vi "MeasureIVandCap.vi"(0 ".NET Refnum in":refnum<k24>, 1 ".NET Refnum":refnum<k24>, 2 "Junction Name":string, 7 "appended path":path, 9 "Numeric":dbl, 12 "new file path (Not A Path if cancelled)":path, 13 "UiDefinition":T1, 14 "Function":string) -> (15 "error out":errorcluster)   [LabVIEW 2020]
uses:
  D:/LabviewDXFViewer/LabviewDXFViewer/bin/Release/LabviewDXFViewer.exe
  LabviewDXFViewer/bin/Release/LabviewDXFViewer.exe
  UIReferences.ctl
  <vilib>/Utility/file.llb/Write Delimited Spreadsheet (DBL).vi
  <vilib>/Utility/file.llb/Write Delimited Spreadsheet (string).vi
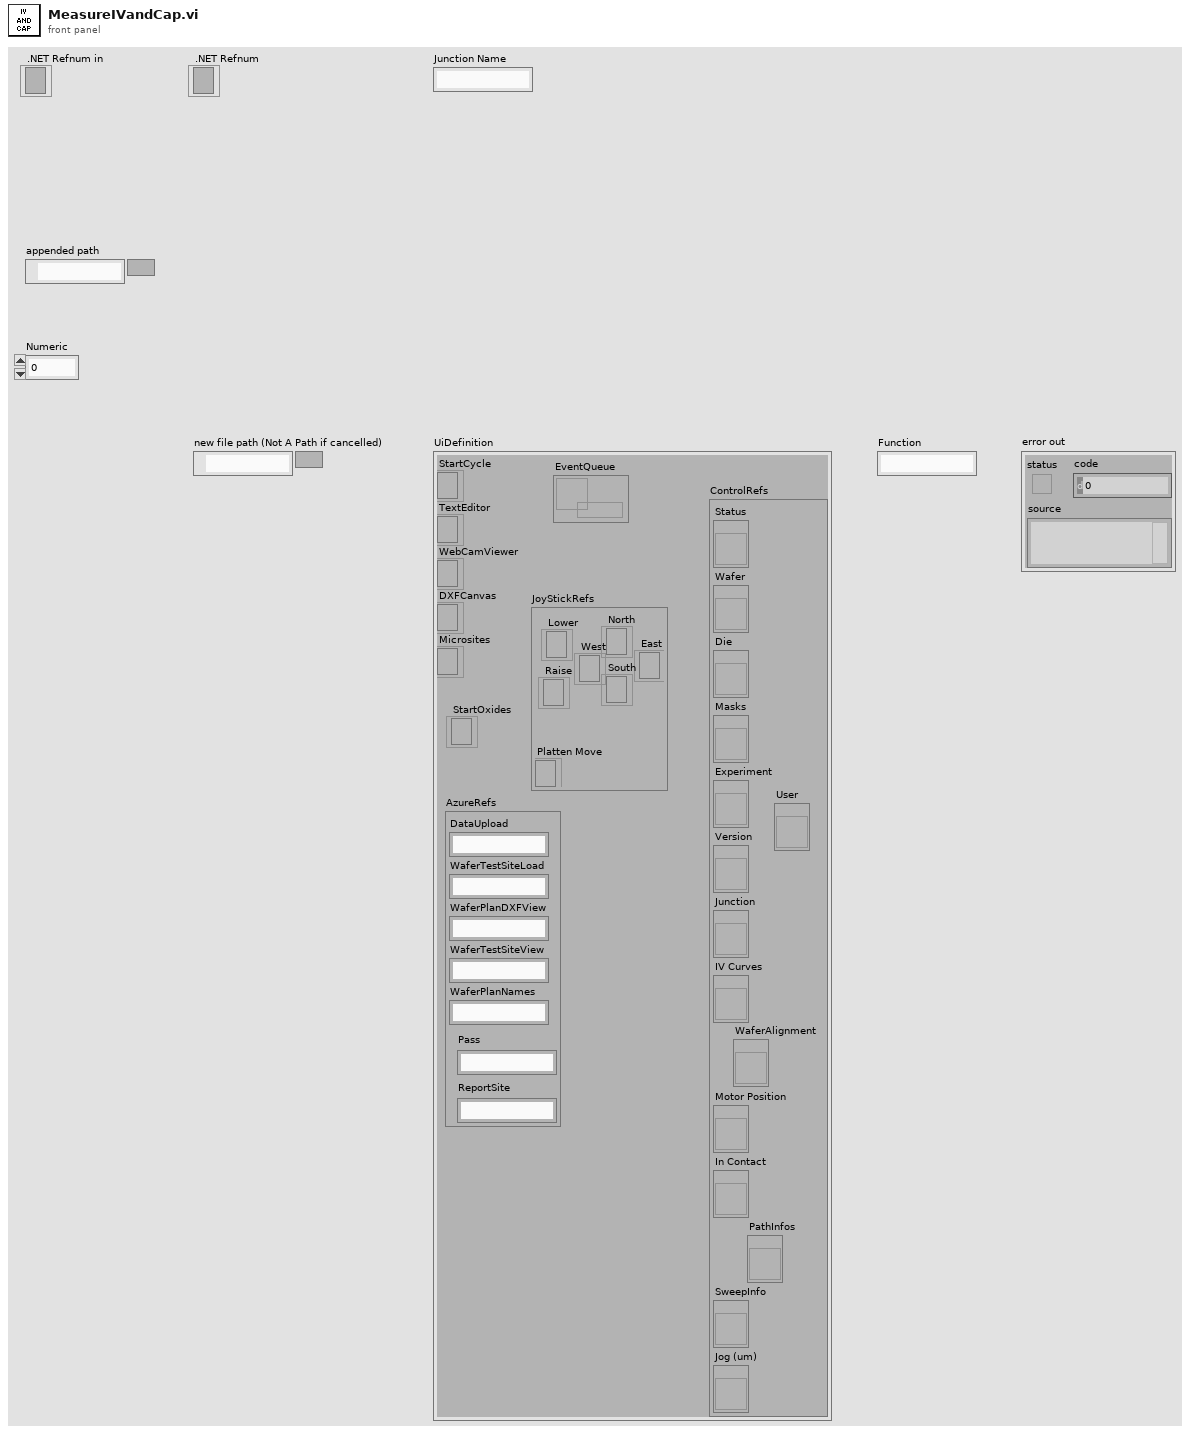
[diagram p1: front panel]
types:
  T1 = typedef "UIReferences.ctl" = cluster{"StartCycle":refnum<k24>, "TextEditor":refnum<k24>, "WebCamViewer":refnum<k24>, "DXFCanvas":refnum<k24>, "Microsites":refnum<k24>, "JoyStickRefs":cluster{"North":refnum<k24>, "Lower":refnum<k24>, "Raise":refnum<k24>, "Platten Move":refnum<k24>, "West":refnum<k24>, "East":refnum<k24>, "South":refnum<k24>}, "AzureRefs":cluster{"DataUpload":string, "WaferTestSiteLoad":string, "WaferPlanDXFView":string, "WaferTestSiteView":string, "WaferPlanNames":string, "Pass":string, "ReportSite":string}, "ControlRefs":cluster{"Status":refnum<vi>, "Wafer":refnum<vi>, "Die":refnum<vi>, "Masks":refnum<vi>, "Experiment":refnum<vi>, "Version":refnum<vi>, "Junction":refnum<vi>, "IV Curves":refnum<vi>, "Motor Position":refnum<vi>, "In Contact":refnum<vi>, "SweepInfo":refnum<vi>, "Jog (um)":refnum<vi>, "PathInfos":refnum<vi>, "User":refnum<vi>, "WaferAlignment":refnum<vi>}, "EventQueue":refnum<queue>, "StartOxides":refnum<k24>}
  T2 = typedef "CapacitanceInfos.ctl" = cluster{"Conductance":dbl, "CapacitanceIV":dbl, "Intercept":dbl, "CapacitanceSW":dbl, "Sum":dbl, "CapacitanceInfos":T3[], "CapacitancePhase":dbl, "dC/dV":dbl, "Function":string}
  T3 = typedef "CapacitanceRecord.ctl" = cluster{"Freq":dbl, "Vpp":dbl, "PhaseS":dbl, "Irms":dbl, "PhaseC":dbl, "Theta":dbl, "VDrive":dbl, "Capacitance":dbl, "Other":dbl}
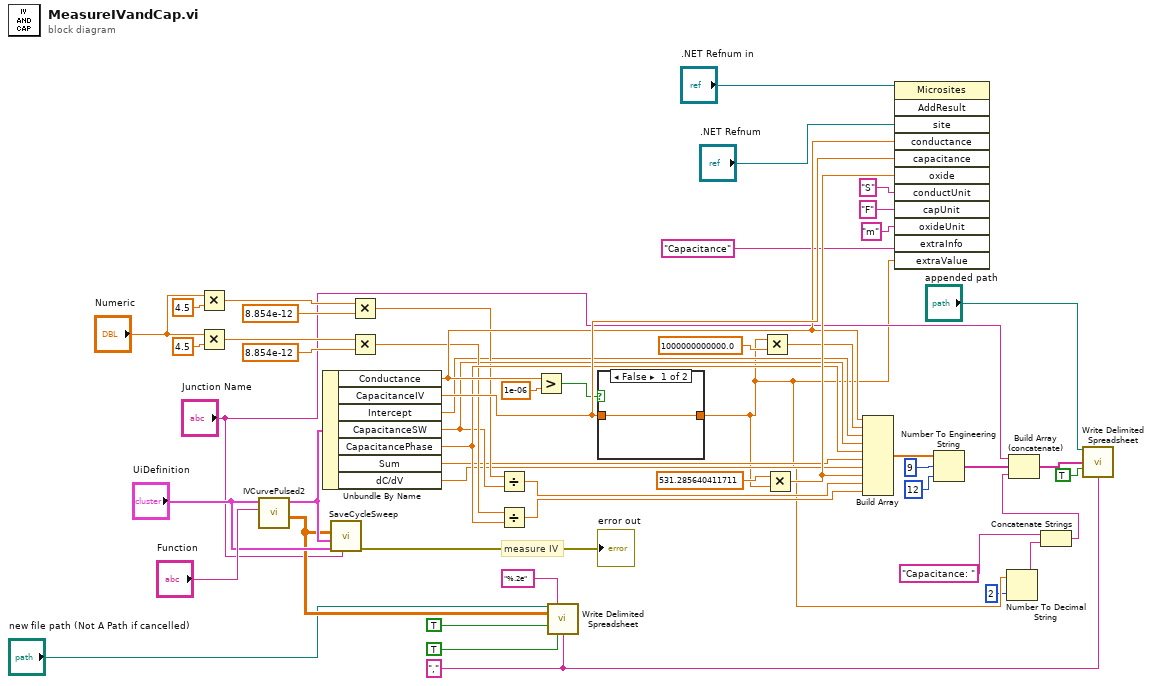
[diagram p0: block diagram]
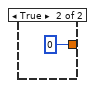
[diagram p2: hidden frame]
diagram:
  w7 = "," ("delimiter (\\t)")
  # "measure IV"
  n1 = Multiply(x="Numeric", y=4.5) -> (x*y=w28:dbl)
  n2 = Multiply(x="Numeric", y=4.5) -> (x*y=w34:dbl)
  n3 = call "IVCurvePulsed2.vi"("Program"="Function", "UiDefinition"="UiDefinition") -> ("appended array"=w18:dbl[][], "InfoCluster"=w48:T2)  [unwired: 8 in]
  n4 = Unbundle By Name(w48) -> ("Conductance"=w50:dbl, "CapacitanceIV"=w51:dbl, "Intercept"=w22:dbl, "CapacitanceSW"=w31:dbl, "CapacitancePhase"=w38:dbl, "Sum"=w23:dbl, "dC/dV"=w24:dbl)
  n5 = call "SaveCycleSweep.vi"("JunctionName"="Junction Name", "UiDefinition 2"="UiDefinition", "InfoCluster"=w48, "appended array"=w18) -> ("error out"=→"error out":errorcluster)  [unwired: 7 in]
  n6 = Multiply(x=w28, y=8.854e-12) -> (x*y=w30:dbl)
  n7 = Multiply(x=w34, y=8.854e-12) -> (x*y=w36:dbl)
  n8 = Divide(x=w30, y=w31) -> (x/y=w32:dbl)
  n9 = Divide(x=w36, y=w38) -> (x/y=w39:dbl)
  n10 = Greater?(x=w50, y=1e-06) -> (0:w40:bool)
  n11 = call-poly <vilib>:"Write Delimited Spreadsheet.vi"("file path (dialog if empty)"="new file path (Not A Path if cancelled)", "format (%.3f)"="%.2e", "2D data"=w18, "append to file? (new file:F)"=TRUE, "transpose? (no:F)"=TRUE, "delimiter (\\t)"=w7) -> ()  [unwired: 8 in, 2 out]
  n12 = case shown="False" w40 {
    tunnel: [w54 0] -> w3
    tunnel: w51 -> [w54 _]
    frame False {
    }
    frame True {
    }
  }
  n13 = Multiply(x=w3, y=1000000000000.0) -> (x*y=w25:dbl)
  n14 = Multiply(x=531.285640411711, y=w3) -> (x*y=w53:dbl)
  n15 = Build Array(w50, w25, w22, w31, w38, w23, w24, w53, w32, w39) -> (w21:dbl[])
  n16 = invoke class="Microsites" method="AddResult"(reference=".NET Refnum in", "site"=".NET Refnum", "conductance"=w50, "capacitance"=w51, "oxide"=w53, "conductUnit"="S", "capUnit"="F", "oxideUnit"="m" ("interceptUnit"), "extraInfo"="Capacitance", "extraValue"=w3) -> ()  [unwired: 2 in, 12 out]
  n17 = Number To Engineering String(2:i16 12 ("precision (6)"), 3:i16 9 ("width (-)"), 4:w21) -> (0:w12:string[])  [unwired: 1 in]
  n18 = Number To Decimal String(number=w3, width (-)=i16 2) -> (decimal integer string=w5:string)
  n19 = Concatenate Strings("Capacitance: ", w5) -> (w1:string)
  n20 = Build Array (concatenate)("Junction Name", w12, w1) -> (w14:string[])
  n21 = call-poly <vilib>:"Write Delimited Spreadsheet.vi"("file path (dialog if empty)"="appended path", "1D data"=w14, "append to file? (new file:F)"=TRUE, "delimiter (\\t)"=w7) -> ()  [unwired: 10 in, 2 out]
